vi "Handle Error.vi"(8 "error in (no error)":errorcluster, 11 "Image Editor Handler in":refnum<class "Image Editor Handler.lvclass">) -> (0 "error out":errorcluster, 2 "Stop Controller":bool, 3 "Image Editor Handler out":refnum<class "Image Editor Handler.lvclass">)   [LabVIEW 2017, in "LV Image Editor Framework.lvlib" / "Image Editor Handler.lvclass"]
uses:
  <vilib>/LIEF/Image Editor Handler/Image Editor Handler.lvclass
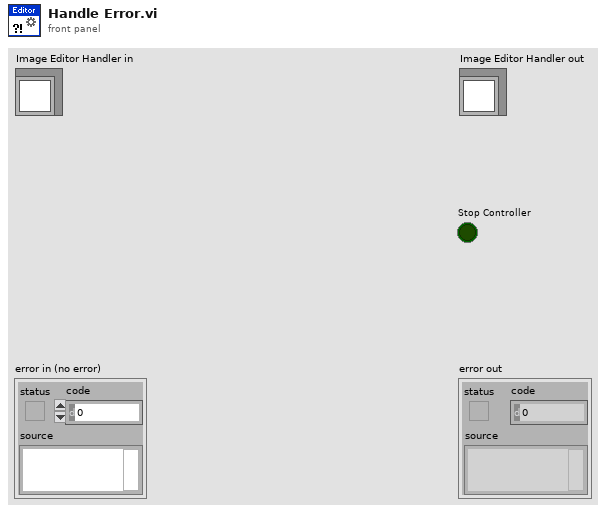
[diagram p1: front panel]
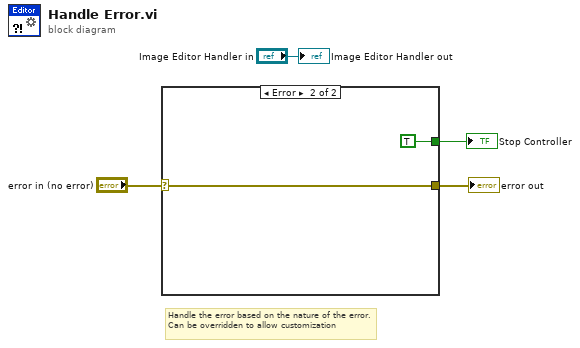
[diagram p0: block diagram]
diagram:
  # "Handle the error based on the nature of the error. Can be overridden to allow customization"
  n1 = case shown="Error" "error in (no error)" {
    selector: "error in (no error)" -> [w5 w7]
    tunnel: [w5 w7] -> w2
    tunnel: [_ TRUE] -> w1
    frame No Error {
    }
    frame Error {
    }
  }
  "error out" <- w2
  "Stop Controller" <- w1
  "Image Editor Handler out" <- "Image Editor Handler in"
